vi "GetPhase.vi"(11 "Frequency":T1) -> (0 "Corrected Theta":dbl, 1 "Omega":dbl format="%.2p", 2 "Simple Theta":dbl)   [LabVIEW 2020]
uses:
  <vilib>/measure/matone.llb/Extract Single Tone Information 1 Chan.vi
  <vilib>/measure/NI_MAPro.lvlib
  <vilib>/measure/NI_MABase.lvlib
panel:
  out "Calculated Phase":dbl
  out "voltage phase":dbl format="%.2p"
  out "detected phase (deg)":dbl
  out "Voltage":waveform(dbl)(graph)
  out "Waveform Graph":waveform(dbl)[](graph)
  out "error out":errorcluster
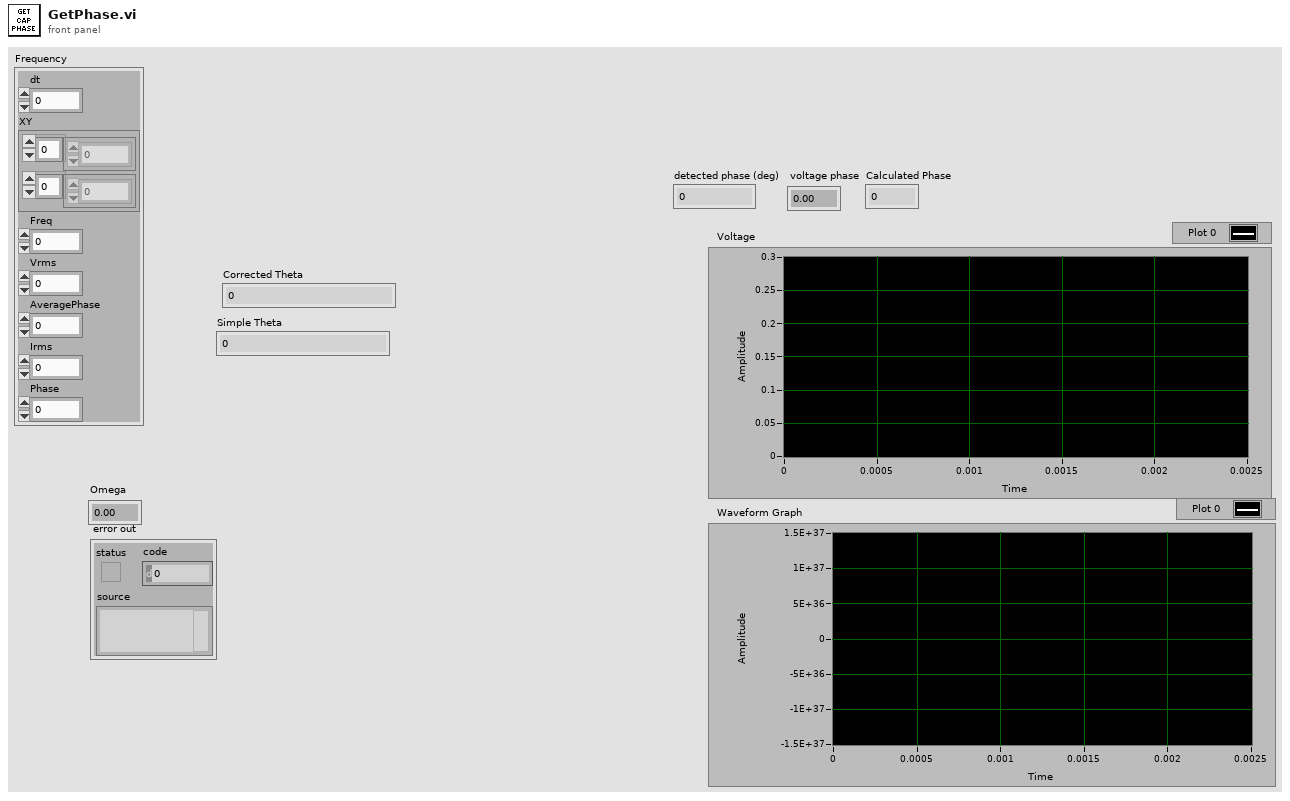
[diagram p1: front panel]
types:
  T1 = cluster{"dt":dbl, "XY":cluster{dbl[], dbl[]}, "Freq":i32, "Vrms":i32, "AveragePhase":i32, "Irms":i32, "Phase":i32}
  T2 = cluster{"approx freq. (optional)":dbl, "search (+/- % of Fsampl.)":dbl}
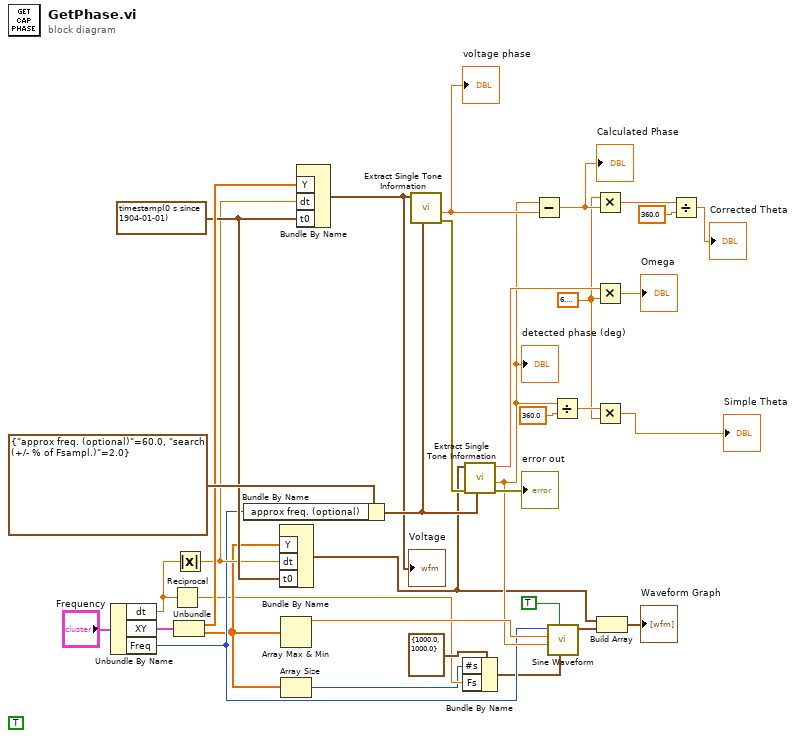
[diagram p0: block diagram]
diagram:
  (unwired) TRUE ("reset signal")
  w15 = 6.283185307179586
  w31 = timestamp(0 s since 1904-01-01) ("t0")
  n1 = Unbundle By Name("Frequency") -> ("dt"=w3:dbl, "XY"=w33:cluster{dbl[], dbl[]}, "Freq"=w10:i32)
  n2 = Reciprocal(x=w3) -> (1/x=w2:dbl)
  n3 = Unbundle(w33) -> (w32:dbl[], w9:dbl[])
  n4 = Absolute Value(x=w3) -> (abs(x)=w21:dbl)
  n5 = Bundle By Name(cluster=T2 {"approx freq. (optional)"=60.0, "search (+/- % of Fsampl.)"=2.0} ("advanced search"), "approx freq. (optional)"=w10) -> (w30:T2)
  n6 = Bundle By Name("Y"=w9, "dt"=w21, "t0"=w31) -> (w6:waveform(dbl))  [unwired: 1 in]
  n7 = Array Max & Min(array=w9) -> (max value=w13:dbl)  [unwired: 3 out]
  n8 = Array Size(array=w9) -> (size(s)=w1:i32)
  n9 = Bundle By Name("Y"=w32, "dt"=w21, "t0"=w31) -> (w20:waveform(dbl))  [unwired: 1 in]
  "Voltage" <- w20
  n10 = call-poly <vilib>:"Extract Single Tone Information.vi"("advanced search"=w30, "time signal in"=w20) -> ("error out"=w24:errorcluster, "detected phase (deg)"=w14:dbl)  [unwired: 4 in, 4 out]
  "voltage phase" <- w14
  n11 = Bundle By Name(cluster=cluster{"Fs":dbl, "#s":dbl} {"Fs"=1000.0, "#s"=1000.0} ("sampling info"), "#s"=w1, "Fs"=w2) -> (w4:cluster{"Fs":dbl, "#s":dbl})
  n12 = call-poly <vilib>:"Extract Single Tone Information.vi"("advanced search"=w30, "error in (no error)"=w24, "time signal in"=w6) -> ("error out"=→"error out":errorcluster, "detected phase (deg)"=w12:dbl, "detected frequency"=w22:dbl)  [unwired: 3 in, 3 out]
  "detected phase (deg)" <- w12
  n13 = Subtract(x=w12, y=w14) -> (x-y=w29:dbl)
  "Calculated Phase" <- w29
  n14 = call <vilib>:"Sine Waveform.vi"("sampling info"=w4, "reset signal"=TRUE, "phase"=w12, "amplitude"=w13, "frequency"=w10) -> ("signal out"=w5:waveform(dbl))  [unwired: 5 in, 1 out]
  n15 = Divide(x=w12, y=360.0) -> (x/y=w18:dbl)
  n16 = Multiply(x=w15, y=w29) -> (x*y=w28:dbl)
  n17 = Multiply(x=w22, y=w15) -> (x*y=→"Omega":dbl)
  n18 = Multiply(x=w18, y=w15) -> (x*y=→"Simple Theta":dbl)
  n19 = Build Array(w6, w5) -> (→"Waveform Graph":waveform(dbl)[])
  n20 = Divide(x=w28, y=360.0) -> (x/y=→"Corrected Theta":dbl)
